vi "ORCA External Trigger with Piezo.vi"() -> ()   [LabVIEW 2012]
uses:
  <vilib>/DAQmx/write.llb/DAQmx Write (Digital Bool 1Line 1Point).vi
  <vilib>/DAQmx/create/channels.llb/DAQmx Create Channel (DO-Digital Output).vi
  <vilib>/DAQmx/write.llb/DAQmx Write (Analog DBL 1Chan 1Samp).vi
  <vilib>/DAQmx/write.llb/DAQmx Write (Digital 1D Bool 1Chan 1Samp).vi
  <vilib>/DAQmx/read.llb/DAQmx Read (Digital Bool 1Line 1Point).vi
  <vilib>/DAQmx/create/channels.llb/DAQmx Create Channel (AO-Voltage-Basic).vi
  <vilib>/DAQmx/read.llb/DAQmx Read (Analog DBL 1Chan 1Samp).vi
  <vilib>/DAQmx/create/channels.llb/DAQmx Create Channel (AI-Voltage-Basic).vi
  <vilib>/Instr/_visa.llb/VISA Configure Serial Port (Instr).vi
  <vilib>/DAQmx/create/channels.llb/DAQmx Create Channel (DI-Digital Input).vi
panel:
  out "Time to next":dbl
  out "Last pos":bool
  out "Waiting":bool
  out "First pos":bool
  out "Pos N":i32
  in  "Positions":i32=1 min=0 max=50 step=1
  in  "Next Pos":bool
  in  "Manual LCVR?":bool
  in  "z offset (um)":dbl=0.29
  in  "use z offset":bool
  in  "Auto Z":bool
  out "Z move":bool
  out "z #":i16
  in  "z step (um)":dbl=0.01
  in  "# z steps":i16=1
  in  "Piezo (um)":dbl format="%#_4g"
  in  "Piezo V":dbl min=0.0 max=10.0 step=0.01 format="%_4g"
  out "Output V":dbl
  in  "Voltages":dbl[][](array[numeric])=[[6.1, 5.6], [1.9, 2.4], [3.3, 3.6]] min=0.0 max=8.0 step=0.1 format="%0.3f"
  in  "LCVR V":dbl min=0.0 max=8.0 step=0.2
  in  "Manual DIO":bool
  in  "Live mode":bool
  out "Duration (s)":dbl
  in  "Int unit":enum16{"ms", "s", "min"}(ring)
  in  "Interval":u32 max=1000 step=1
  in  "Stop acq":bool
  in  "Exposure (ms)":u32=50 min=1 max=2000 step=5
  out "Ch N":T1
  in  "Ch 2":T2(radio)=enum."Radio Selection 3"
  out "Ch":enum32{"0", "1", "2"}(radio)
  in  "Ch 1":T2(radio)=enum."Radio Selection 2"
  in  "Ch 0":T2(radio)
  out "Current Frame":i32
  out "Total Frames":i16
  in  "Frames":i16=1
  in  "Channels":i16=1 min=1 max=3 step=1
  in  "SIM \nFrames":i16=9
  in  "stop":bool
  in  "Acquire":bool
  # "LCVR Voltage Settings"
  # "Voltage #"
  # "Channel #"
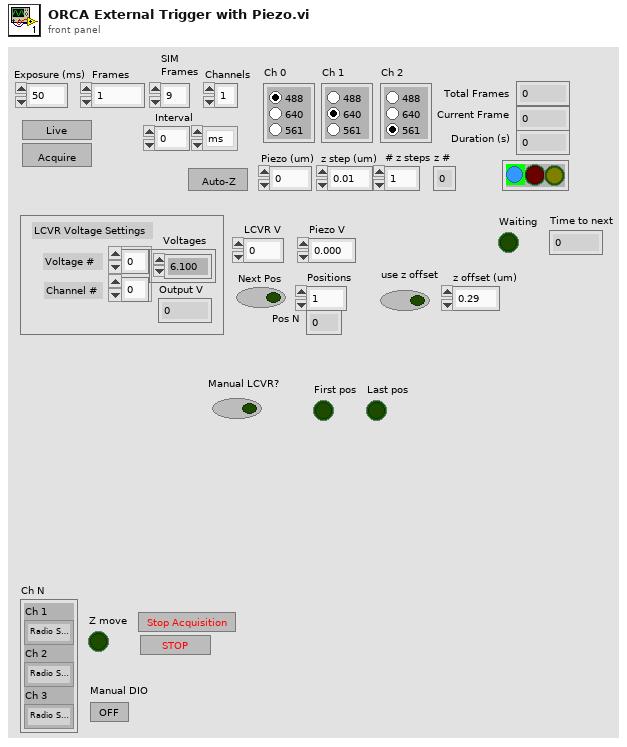
[diagram p1: front panel]
types:
  T1 = cluster{"Ch 1":enum32{"Radio Selection 1", "Radio Selection 2", "Radio Selection 3"}, "Ch 2":enum32{"Radio Selection 1", "Radio Selection 2", "Radio Selection 3"}, "Ch 3":enum32{"Radio Selection 1", "Radio Selection 2", "Radio Selection 3"}}
  T2 = enum32{"Radio Selection 1", "Radio Selection 2", "Radio Selection 3"}
  T3 = cluster{"Ch 0":enum32{"Radio Selection 1", "Radio Selection 2", "Radio Selection 3"}, "Ch 1":enum32{"Radio Selection 1", "Radio Selection 2", "Radio Selection 3"}, "Ch 2":enum32{"Radio Selection 1", "Radio Selection 2", "Radio Selection 3"}}
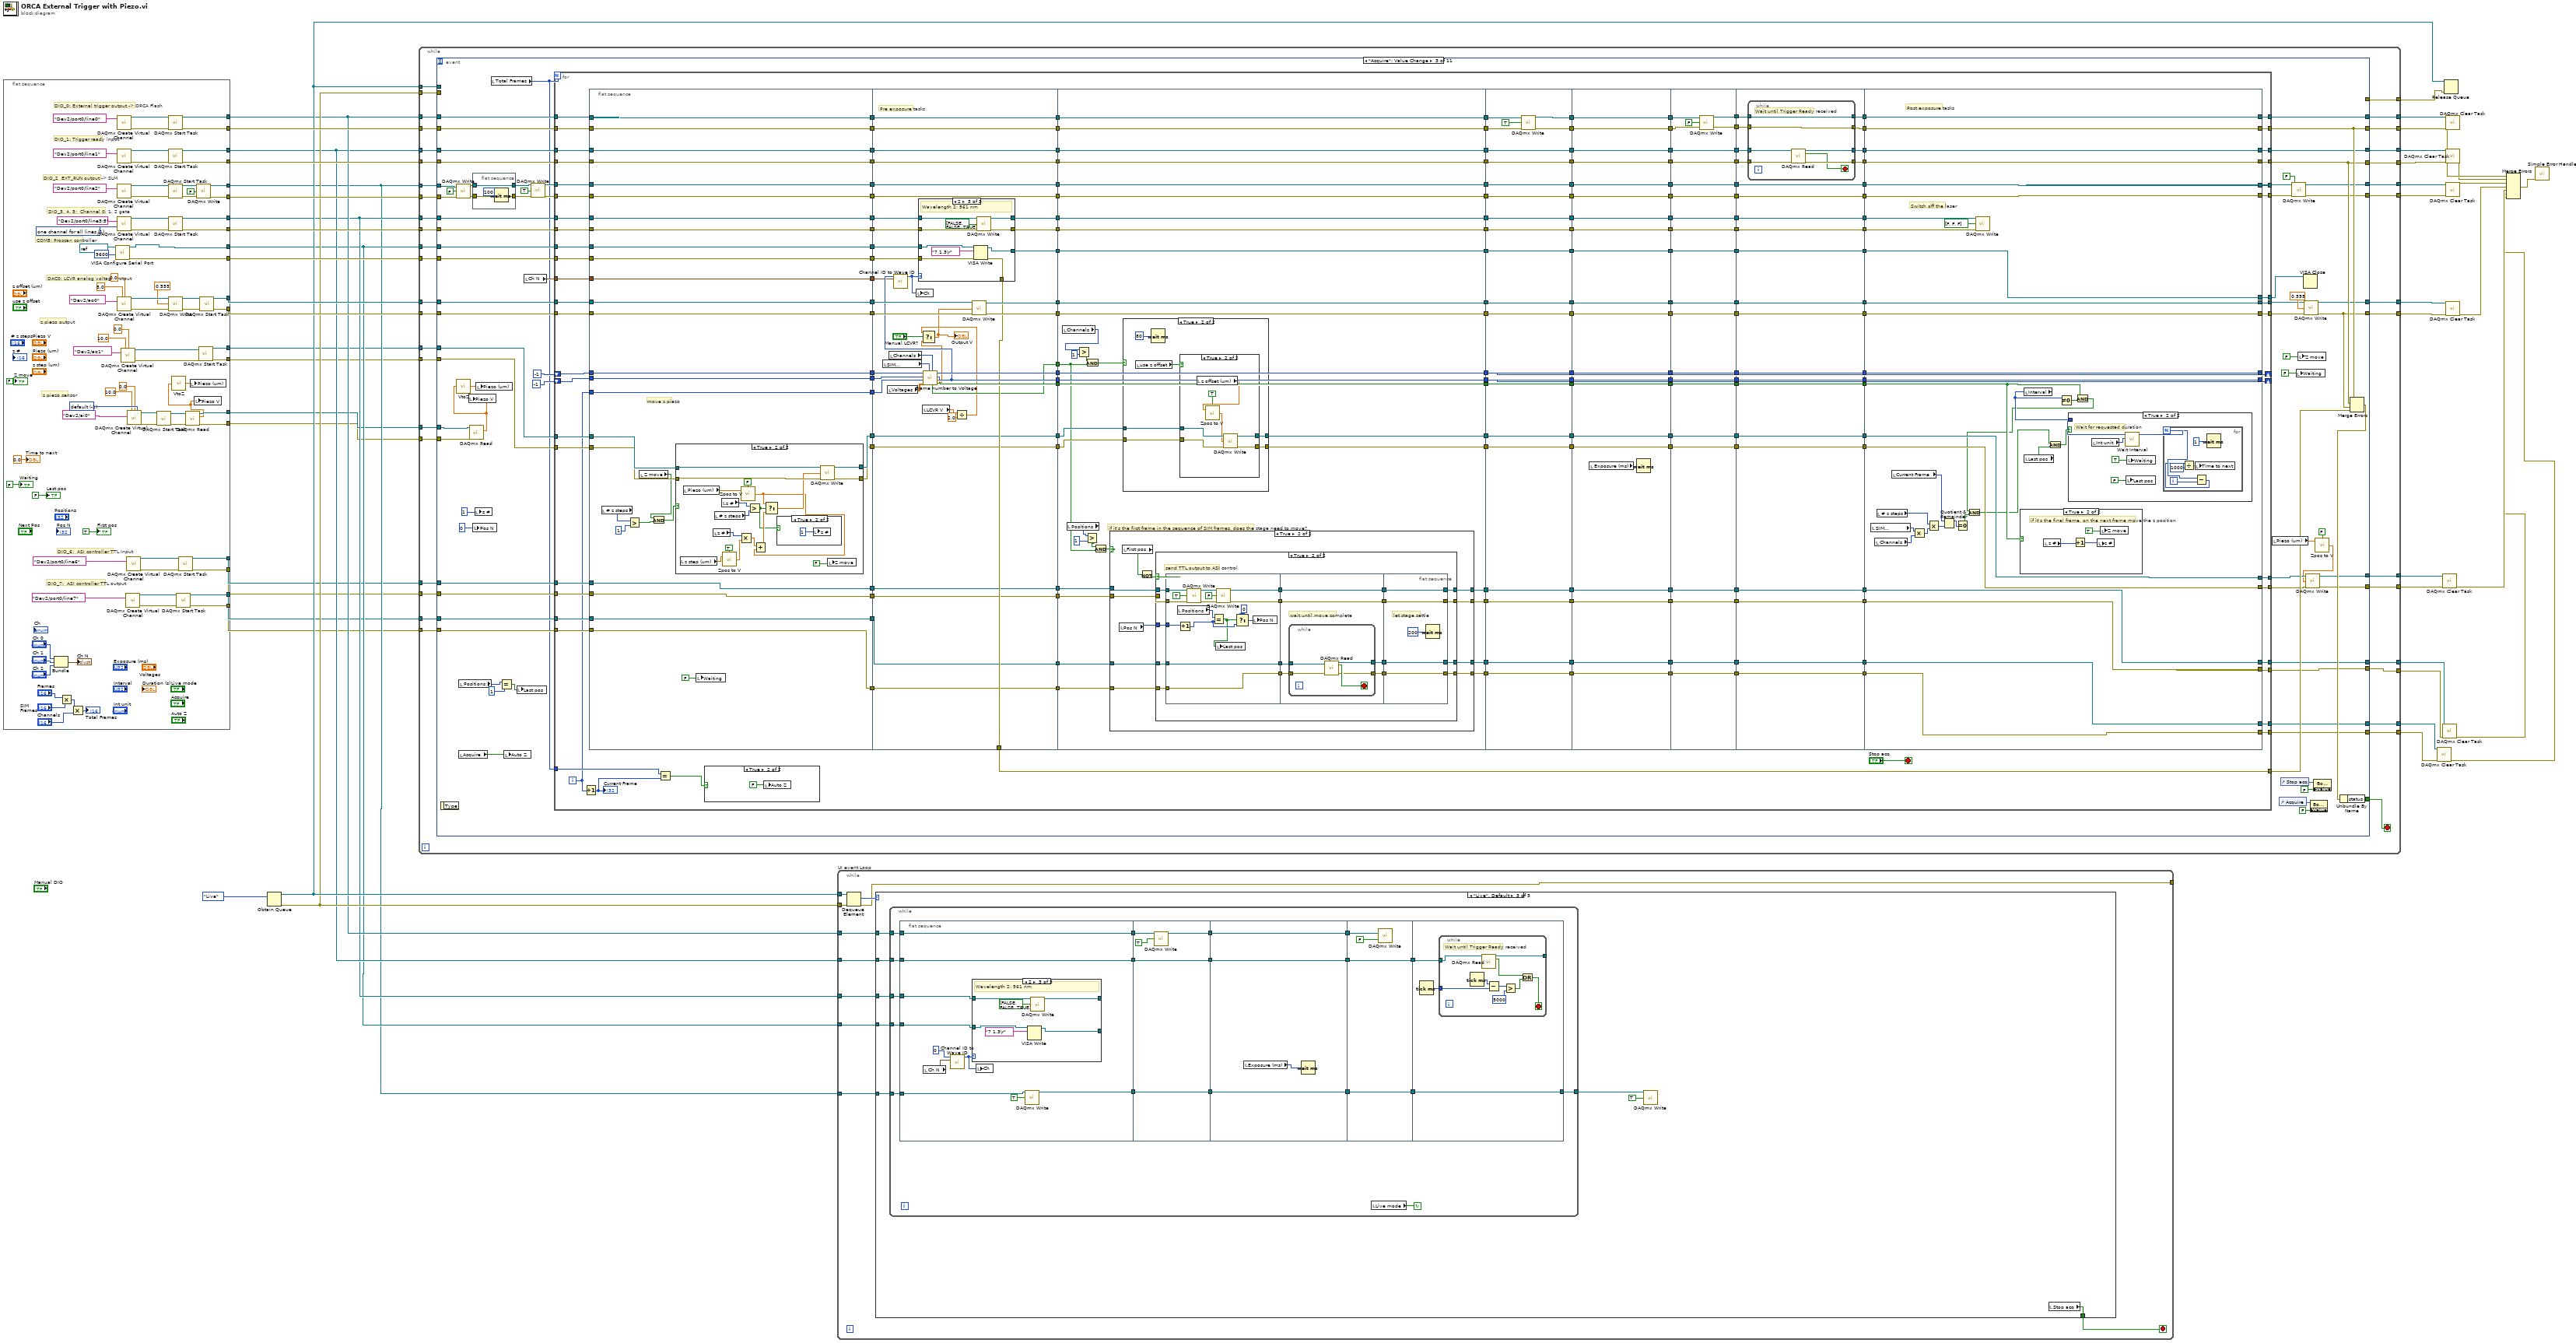
[diagram p0: block diagram]
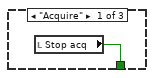
[diagram p2: hidden frame]
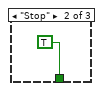
[diagram p3: hidden frame]
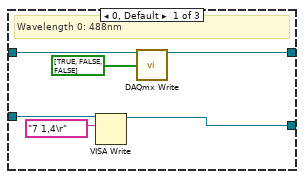
[diagram p4: hidden frame]
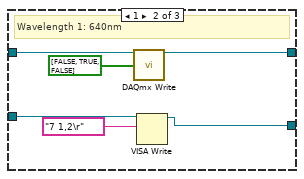
[diagram p5: hidden frame]
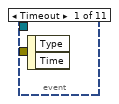
[diagram p6: hidden frame]
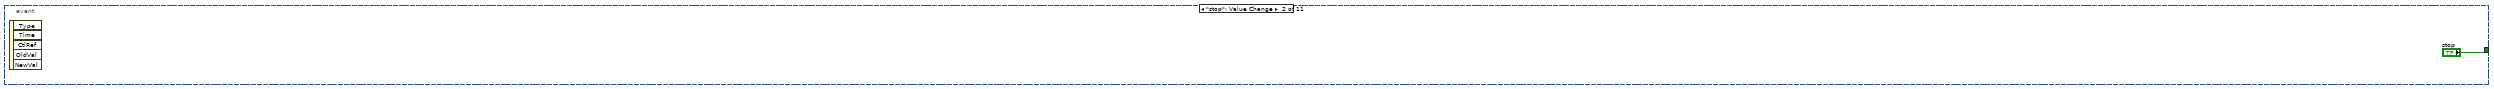
[diagram p7: hidden frame]
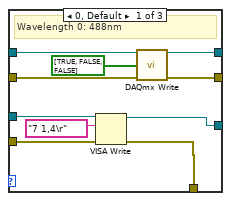
[diagram p11: hidden frame]
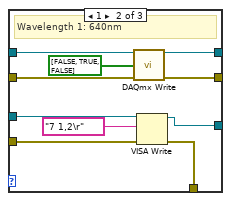
[diagram p12: hidden frame]
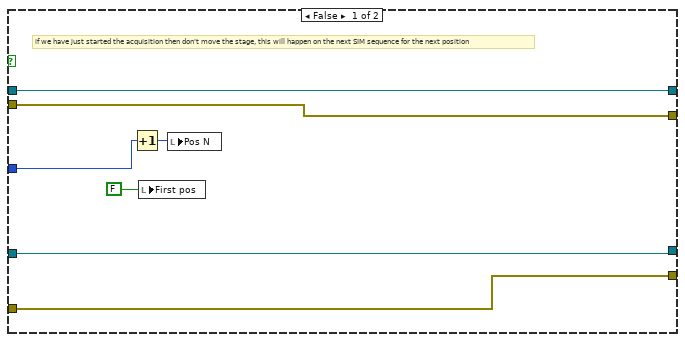
[diagram p14: hidden frame]
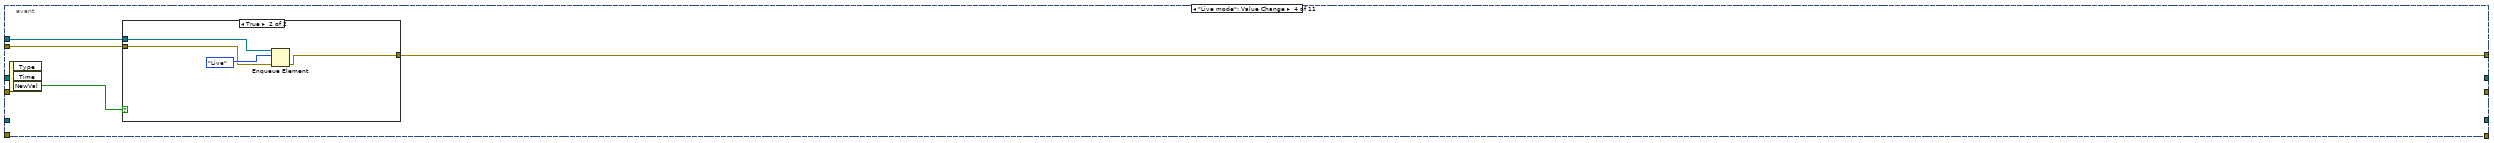
[diagram p19: hidden frame]
diagram:
  n1 = flat-sequence {
    tunnel: [w124] -> w22
    tunnel: [w123] -> w45
    tunnel: [w119] -> w21
    tunnel: [w118] -> w43
    tunnel: [w104] -> w40
    tunnel: [w103] -> w39
    tunnel: [w94] -> w18
    tunnel: [w93] -> w33
    tunnel: [w92] -> w20
    tunnel: [w91] -> w28
    tunnel: [w82] -> w19
    tunnel: [w81] -> w27
    tunnel: [w64] -> w17
    tunnel: [w65] -> w16
    tunnel: [w71] -> w15
    tunnel: [w70] -> w14
    tunnel: [w57] -> w10
    tunnel: [w56] -> w9
    tunnel: [w51] -> w5
    tunnel: [w50] -> w4
    frame #0 {
      w74 = -1 items=["default"=-1, "RSE"=10083, "NRSE"=10078, "Differential"=10106, "Pseudodifferential"=12529] ("input terminal configuration")
      w89 = 1 items=["one channel for each line", "one channel for all lines"] ("line grouping")
      # "DIO_7:  ASI controller TTL output"
      # "DIO_6:  ASI controller TTL Input"
      # "z piezo sensor"
      # "z piezo output"
      # "COM5: Proscan controller"
      # "DIO_3, 4, 5:  Channel 0, 1, 2 gate"
      # "DIO_2  EXT_RUN output -> SLM"
      # "DAC0: LCVR analog voltage output"
      # "DIO_1: Trigger ready input"
      # "DIO_0: External trigger output -> ORCA Flash"
      n2 = Bundle("Ch 0"="Ch 0", "Ch 1"="Ch 1", "Ch 2"="Ch 2") -> (→"Ch N":T3)  [unwired: 1 in]
      n3 = Multiply(x="Frames", y="SIM \nFrames") -> (x*y=w115:i16)
      n4 = Multiply(x=w115, y="Channels") -> (x*y=→"Total Frames":i16)
      n5 = call-poly "VISA Configure Serial Port"("VISA resource name"=refnum<visa-resource-name> "COM5", "baud rate (9600)"=u32 9600) -> ("VISA resource name out"=w82:refnum<visa-resource-name>, "error out"=w81:errorcluster)  [unwired: 12 in]
      n6 = call-poly <vilib>:"DAQmx Create Virtual Channel.vi"("lines"=tag "Dev2/port0/line0") -> ("task out"=w126:refnum<k21>, "error out"=w127:errorcluster)  [unwired: 13 in]
      n7 = call-poly <vilib>:"DAQmx Create Virtual Channel.vi"("lines"=tag "Dev2/port0/line1") -> ("task out"=w121:refnum<k21>, "error out"=w120:errorcluster)  [unwired: 13 in]
      n8 = call-poly <vilib>:"DAQmx Create Virtual Channel.vi"("lines"=tag "Dev2/port0/line2") -> ("task out"=w101:refnum<k21>, "error out"=w100:errorcluster)  [unwired: 13 in]
      n9 = call-poly <vilib>:"DAQmx Create Virtual Channel.vi"("lines"="Dev2/port0/line3:5", "line grouping"=w89) -> ("task out"=w99:refnum<k21>, "error out"=w98:errorcluster)  [unwired: 12 in]
      n10 = call-poly <vilib>:"DAQmx Create Virtual Channel.vi"("maximum value"=5.0, "minimum value"=0.0, "physical channels"=tag "Dev2/ao0") -> ("task out"=w107:refnum<k21>, "error out"=w106:errorcluster)  [unwired: 11 in]
      n11 = call-poly <vilib>:"DAQmx Create Virtual Channel.vi"("maximum value"=10.0, "minimum value"=0.0, "physical channels"=tag "Dev2/ao1") -> ("task out"=w77:refnum<k21>, "error out"=w76:errorcluster)  [unwired: 11 in]
      n12 = call-poly <vilib>:"DAQmx Create Virtual Channel.vi"("lines"=tag "Dev2/port0/line7") -> ("task out"=w53:refnum<k21>, "error out"=w52:errorcluster)  [unwired: 13 in]
      n13 = call-poly <vilib>:"DAQmx Create Virtual Channel.vi"("lines"=tag "Dev2/port0/line6") -> ("task out"=w59:refnum<k21>, "error out"=w58:errorcluster)  [unwired: 13 in]
      n14 = call-poly <vilib>:"DAQmx Create Virtual Channel.vi"("maximum value"=10.0, "minimum value"=0.0, "input terminal configuration"=w74, "physical channels"=tag "Dev2/ai0" ("Physical Channel")) -> ("task out"=w69:refnum<k21>, "error out"=w68:errorcluster)  [unwired: 10 in]
      n15 = call <vilib>:"DAQmx Start Task.vi"("task/channels in"=w69, "error in"=w68) -> ("task out"=w67:refnum<k21>, "error out"=w66:errorcluster)  [unwired: 12 in]
      n16 = call <vilib>:"DAQmx Start Task.vi"("task/channels in"=w126, "error in"=w127) -> ("task out"=w124:refnum<k21>, "error out"=w123:errorcluster)  [unwired: 12 in]
      n17 = call <vilib>:"DAQmx Start Task.vi"("task/channels in"=w121, "error in"=w120) -> ("task out"=w119:refnum<k21>, "error out"=w118:errorcluster)  [unwired: 12 in]
      n18 = call <vilib>:"DAQmx Start Task.vi"("task/channels in"=w101, "error in"=w100) -> ("task out"=w97:refnum<k21>, "error out"=w96:errorcluster)  [unwired: 12 in]
      n19 = call <vilib>:"DAQmx Start Task.vi"("task/channels in"=w99, "error in"=w98) -> ("task out"=w92:refnum<k21>, "error out"=w91:errorcluster)  [unwired: 12 in]
      n20 = call-poly <vilib>:"DAQmx Write.vi"("task/channels in"=w107, "data"=0.555, "error in"=w106) -> ("task out"=w111:refnum<k21>, "error out"=w110:errorcluster)  [unwired: 10 in, 1 out]
      n21 = call <vilib>:"DAQmx Start Task.vi"("task/channels in"=w53, "error in"=w52) -> ("task out"=w51:refnum<k21>, "error out"=w50:errorcluster)  [unwired: 12 in]
      n22 = call <vilib>:"DAQmx Start Task.vi"("task/channels in"=w59, "error in"=w58) -> ("task out"=w57:refnum<k21>, "error out"=w56:errorcluster)  [unwired: 12 in]
      n23 = call-poly <vilib>:"DAQmx Read.vi"("task/channels in"=w67, "error in"=w66) -> ("task out"=w64:refnum<k21>, "data"=w61:dbl, "error out"=w65:errorcluster)  [unwired: 11 in]
      n24 = call "VtoZ.vi"("Voltage IN"=w61) -> ("Zpos OUT (um)"=w62:dbl)
      n25 = local write "Piezo (um)"(w62) -> ()
      n26 = local write "Piezo V"(w61) -> ()
      n27 = call-poly <vilib>:"DAQmx Write.vi"("task/channels in"=w97, "data"=FALSE, "error in"=w96) -> ("task out"=w94:refnum<k21>, "error out"=w93:errorcluster)  [unwired: 10 in, 1 out]
      n28 = call <vilib>:"DAQmx Start Task.vi"("task/channels in"=w77, "error in"=w76) -> ("task out"=w71:refnum<k21>, "error out"=w70:errorcluster)  [unwired: 12 in]
      n29 = call <vilib>:"DAQmx Start Task.vi"("task/channels in"=w111, "error in"=w110) -> ("task out"=w104:refnum<k21>, "error out"=w103:errorcluster)  [unwired: 12 in]
      "Z move" <- FALSE ("Z move")
      "First pos" <- TRUE ("First pos")
      "Waiting" <- FALSE ("Waiting")
      "Last pos" <- FALSE ("Last pos")
      "Time to next" <- 0.0 ("Time to next")
    }
  }
  n30 = Obtain Queue(element data type=enum16{"Live", "Stop", "Acquire"}."Live") -> (queue out=w25:refnum<queue>, error out=w23:errorcluster)  [unwired: 4 in, 1 out]
  n31 = while {
    tunnel: w22 -> [w164]
    tunnel: [w163] -> w46
    tunnel: w45 -> [w162]
    tunnel: [w161] -> w44
    tunnel: w21 -> [w160]
    tunnel: w43 -> [w159]
    tunnel: [w158] -> w42
    tunnel: [w157] -> w41
    tunnel: w40 -> [w156]
    tunnel: w39 -> [w155]
    tunnel: [w154] -> w35
    tunnel: [w153] -> w34
    tunnel: w18 -> [w152]
    tunnel: w33 -> [w151]
    tunnel: [w150] -> w29
    tunnel: [w149] -> w31
    tunnel: w20 -> [w148]
    tunnel: w28 -> [w147]
    tunnel: w19 -> [w146]
    tunnel: w27 -> [w145]
    tunnel: w25 -> [w144]
    tunnel: [w143] -> w24
    tunnel: w23 -> [w142]
    tunnel: w17 -> [w141]
    tunnel: w16 -> [w140]
    tunnel: w15 -> [w139]
    tunnel: w14 -> [w138]
    tunnel: [w137] -> w13
    tunnel: [w136] -> w12
    tunnel: w10 -> [w135]
    tunnel: w9 -> [w134]
    tunnel: [w133] -> w7
    tunnel: [w132] -> w6
    tunnel: w5 -> [w131]
    tunnel: w4 -> [w130]
    tunnel: [w129] -> w2
    tunnel: [w128] -> w1
    stop <- w165 stop-if-true
    n32 = event shown="[2] \"Acquire\": Value Change" {
      selector: _ -> [_ _ _ _ _ _ _ _ _ _ _]
      dyn-events: _ -> [_ _ _ _ _ _ _ _ _ _ _]
      timeout: _ -> [_ _ _ _ _ _ _ _ _ _ _]
      tunnel: [_ "stop" w241 _ _ _ _ _ _ _ _] -> w165
      tunnel: w164 -> [_ _ w240 _ _ _ _ _ _ _ _]
      tunnel: [_ _ w238 _ _ _ _ _ _ _ _] -> w163
      tunnel: w162 -> [_ _ w239 _ _ _ _ _ _ _ _]
      tunnel: [_ _ w232 _ _ _ _ _ _ _ _] -> w161
      tunnel: w160 -> [_ _ w235 _ _ _ _ _ _ _ _]
      tunnel: w159 -> [_ _ w234 _ _ _ _ _ _ _ _]
      tunnel: [_ _ w231 _ _ _ _ _ _ _ _] -> w158
      tunnel: [_ _ w230 _ _ _ _ _ _ _ _] -> w157
      tunnel: w156 -> [_ _ w227 _ _ w858 _ _ _ _ _]
      tunnel: w155 -> [_ _ w226 _ _ w857 _ _ _ _ _]
      tunnel: [_ _ w222 _ _ _ _ _ _ _ _] -> w154
      tunnel: [_ _ w221 _ _ _ _ _ _ _ _] -> w153
      tunnel: w152 -> [_ _ w202 _ _ _ _ _ _ _ _]
      tunnel: w151 -> [_ _ w201 _ _ _ _ _ _ _ _]
      tunnel: [_ _ w204 _ _ _ _ _ _ _ _] -> w150
      tunnel: [_ _ w206 _ _ _ _ _ _ _ _] -> w149
      tunnel: w148 -> [_ _ w217 _ w838 _ _ _ _ _ _]
      tunnel: w147 -> [_ _ w216 _ w837 _ _ _ _ _ _]
      tunnel: w146 -> [_ _ w212 _ _ _ _ _ _ _ _]
      tunnel: w145 -> [_ _ w211 _ _ _ _ _ _ _ _]
      tunnel: w144 -> [_ _ _ w827 _ _ _ _ _ _ _]
      tunnel: [_ _ _ w826 _ _ _ _ _ _ _] -> w143
      tunnel: w142 -> [_ _ _ w825 _ _ _ _ _ _ _]
      tunnel: w141 -> [_ _ w196 _ _ _ _ _ _ w893 _]
      tunnel: w140 -> [_ _ w195 _ _ _ _ _ _ w892 _]
      tunnel: w139 -> [_ _ w194 _ _ _ _ _ w885 w891 _]
      tunnel: w138 -> [_ _ w193 _ _ _ _ _ w884 w888 _]
      tunnel: [_ _ w188 _ _ _ _ _ _ _ _] -> w137
      tunnel: [_ _ w187 _ _ _ _ _ _ _ _] -> w136
      tunnel: w135 -> [_ _ w181 _ _ _ _ _ _ _ w913]
      tunnel: w134 -> [_ _ w180 _ _ _ _ _ _ _ w912]
      tunnel: [_ _ w178 _ _ _ _ _ _ _ _] -> w133
      tunnel: [_ _ w177 _ _ _ _ _ _ _ _] -> w132
      tunnel: w131 -> [_ _ w176 _ _ _ _ _ _ _ _]
      tunnel: w130 -> [_ _ w175 _ _ _ _ _ _ _ _]
      tunnel: [_ _ w174 _ _ _ _ _ _ _ _] -> w129
      tunnel: [_ _ w173 _ _ _ _ _ _ _ _] -> w128
      event Timeout {
        n33 = event-data() -> ()  [unwired: 1 in, 2 out]
      }
      event "stop": Value Change {
        n34 = event-data() -> ()  [unwired: 1 in, 5 out]
      }
      event "Acquire": Value Change {
        n35 = event-data() -> ()  [unwired: 1 in, 1 out]
        n36 = call-poly <vilib>:"DAQmx Write.vi"("task/channels in"=w202, "data"=FALSE, "error in"=w201) -> ("task out"=w197:refnum<k21>, "error out"=w199:errorcluster)  [unwired: 10 in, 1 out]
        n37 = local read "Acquire"() -> (w168:bool)
        n38 = local read "Positions"() -> (w171:i32)
        n39 = call-poly <vilib>:"DAQmx Read.vi"("task/channels in"=w196, "error in"=w195) -> ("data"=w185:dbl)  [unwired: 11 in, 2 out]
        n40 = call "VtoZ.vi"("Voltage IN"=w185) -> ("Zpos OUT (um)"=w186:dbl)
        n41 = local write "Piezo V"(w185) -> ()
        n42 = local write "Pos N"(0 ("Pos N")) -> ()
        n43 = flat-sequence {
          tunnel: [w244] -> w200
          tunnel: w199 -> [w244]
          tunnel: [w243] -> w198
          tunnel: w197 -> [w243]
          frame #0 {
            n44 = Wait (ms)(milliseconds to wait=u32 100) -> ()  [unwired: 1 out]
          }
        }
        n45 = local write "z #"(i16 1 ("z #")) -> ()
        n46 = local write "Piezo (um)"(w186) -> ()
        n47 = local read "Total Frames"() -> (w167:i16)
        n48 = Equal?(x=w171, y=1) -> (x = y?=w169:bool)
        n49 = local write "Auto Z"(w168) -> ()
        n50 = local write "Last pos"(w169) -> ()
        n51 = local read "Ch N"() -> (w215:T1)
        n52 = call-poly <vilib>:"DAQmx Write.vi"("task/channels in"=w198, "data"=TRUE, "error in"=w200) -> ("task out"=w219:refnum<k21>, "error out"=w218:errorcluster)  [unwired: 10 in, 1 out]
        n53 = for {
          N: w167 -> [_]
          tunnel: w240 -> [w431]
          tunnel: w239 -> [w430]
          tunnel: [w428] -> w238
          tunnel: [w427] -> w232
          tunnel: w235 -> [w425]
          tunnel: w234 -> [w423]
          tunnel: [w422] -> w231
          tunnel: [w421] -> w230
          shift-right: [w417] -> _
          shift-left: i16 -1 ("Voltage out") -> [w419]
          shift-right: [w415] -> _
          shift-left: i16 -1 ("Channel out") -> [w418]
          tunnel: w227 -> [w413]
          tunnel: w226 -> [w412]
          tunnel: [w411] -> w224
          tunnel: [w409] -> w223
          tunnel: [w399] -> w207
          tunnel: w219 -> [w396]
          tunnel: [w395] -> w205
          tunnel: w218 -> [w392]
          tunnel: w217 -> [w391]
          tunnel: w216 -> [w390]
          tunnel: w215 -> [w389]
          tunnel: w212 -> [w355]
          tunnel: w211 -> [w354]
          tunnel: [w353] -> w209
          tunnel: [w348] -> w210
          tunnel: w194 -> [w302]
          tunnel: w193 -> [w301]
          tunnel: [w293] -> w190
          tunnel: [w289] -> w189
          tunnel: w181 -> [w284]
          tunnel: w180 -> [w283]
          tunnel: [w268] -> w178
          tunnel: [w267] -> w177
          tunnel: w176 -> [w266]
          tunnel: w175 -> [w265]
          tunnel: [w250] -> w174
          tunnel: [w249] -> w173
          tunnel: w167 -> [w248]
          i -> [w246]
          stop <- "Stop acq" stop-if-true
          n54 = Increment(x=w246) -> (x+1=w245:i32)
          "Current Frame" <- w245
          n55 = flat-sequence {
            tunnel: w354 -> [w447]
            tunnel: w355 -> [w448]
            tunnel: w389 -> [w449]
            tunnel: w390 -> [w450]
            tunnel: w391 -> [w451]
            tunnel: w392 -> [w452]
            tunnel: w396 -> [w453]
            tunnel: w412 -> [w454]
            tunnel: w413 -> [w455]
            tunnel: w418 -> [w456]
            tunnel: w419 -> [w457]
            tunnel: w246 -> [w458]
            tunnel: w423 -> [w459]
            tunnel: w425 -> [w460]
            tunnel: w430 -> [w461]
            tunnel: w431 -> [w462]
            tunnel: [w462] -> w318
            tunnel: [w461] -> w317
            tunnel: [w460] -> w316
            tunnel: [w459] -> w315
            tunnel: [w458] -> w314
            tunnel: [w457] -> w313
            tunnel: [w456] -> w312
            tunnel: [w455] -> w311
            tunnel: [w454] -> w310
            tunnel: [w453] -> w309
            tunnel: [w452] -> w308
            tunnel: [w451] -> w307
            tunnel: [w450] -> w306
            tunnel: [w449] -> w305
            tunnel: [w448] -> w304
            tunnel: [w447] -> w303
            tunnel: w302 -> [w446]
            tunnel: w301 -> [w445]
            tunnel: [w439] -> w297
            tunnel: [w438] -> w294
            tunnel: w284 -> [w437]
            tunnel: w283 -> [w436]
            tunnel: [w437] -> w281
            tunnel: [w436] -> w279
            tunnel: w266 -> [w435]
            tunnel: w265 -> [w434]
            tunnel: [w435] -> w263
            tunnel: [w434] -> w261
            tunnel: [w525] -> w347
            tunnel: [w524] -> w345
            tunnel: [w523] -> w343
            tunnel: [w522] -> w341
            tunnel: [w516] -> w339
            tunnel: [w506] -> w337
            tunnel: [w512] -> w335
            tunnel: [w511] -> w333
            tunnel: [w510] -> w331
            tunnel: [w509] -> w329
            tunnel: [w503] -> w327
            tunnel: [w502] -> w325
            tunnel: [w501] -> w323
            tunnel: [w498] -> w321
            tunnel: [w497] -> w348
            tunnel: [w496] -> w319
            tunnel: w318 -> [w525]
            tunnel: w317 -> [w524]
            tunnel: w316 -> [w523]
            tunnel: w315 -> [w522]
            tunnel: w314 -> [w517]
            tunnel: w313 -> [w519]
            tunnel: w312 -> [w518]
            tunnel: w311 -> [w514]
            tunnel: w310 -> [w513]
            tunnel: w309 -> [w510]
            tunnel: w308 -> [w509]
            tunnel: w307 -> [w508]
            tunnel: w306 -> [w507]
            tunnel: w305 -> [w504]
            tunnel: w304 -> [w500]
            tunnel: w303 -> [w499]
            tunnel: [w495] -> w298
            tunnel: w297 -> [w495]
            tunnel: [w494] -> w295
            tunnel: w294 -> [w494]
            tunnel: [w487] -> w282
            tunnel: w281 -> [w487]
            tunnel: [w486] -> w280
            tunnel: w279 -> [w486]
            tunnel: [w485] -> w264
            tunnel: w263 -> [w485]
            tunnel: [w484] -> w262
            tunnel: w261 -> [w484]
            tunnel: w347 -> [w590]
            tunnel: [w590] -> w346
            tunnel: w345 -> [w589]
            tunnel: [w589] -> w344
            tunnel: w343 -> [w588]
            tunnel: [w588] -> w342
            tunnel: w341 -> [w587]
            tunnel: [w587] -> w340
            tunnel: w339 -> [w586]
            tunnel: [w586] -> w338
            tunnel: w337 -> [w585]
            tunnel: [w585] -> w336
            tunnel: w335 -> [w584]
            tunnel: [w584] -> w334
            tunnel: w333 -> [w583]
            tunnel: [w583] -> w332
            tunnel: w331 -> [w582]
            tunnel: [w582] -> w330
            tunnel: w329 -> [w581]
            tunnel: [w581] -> w328
            tunnel: w327 -> [w580]
            tunnel: [w580] -> w326
            tunnel: w325 -> [w579]
            tunnel: [w579] -> w324
            tunnel: w323 -> [w578]
            tunnel: [w578] -> w322
            tunnel: w321 -> [w577]
            tunnel: [w577] -> w320
            tunnel: w319 -> [w568]
            tunnel: [w570] -> w299
            tunnel: w298 -> [w572]
            tunnel: w295 -> [w571]
            tunnel: [w569] -> w285
            tunnel: w282 -> [w564]
            tunnel: w280 -> [w563]
            tunnel: [w561] -> w274
            tunnel: [w560] -> w269
            tunnel: w264 -> [w559]
            tunnel: w262 -> [w558]
            tunnel: [w557] -> w256
            tunnel: [w556] -> w251
            tunnel: [w698] -> w388
            tunnel: [w697] -> w386
            tunnel: [w696] -> w384
            tunnel: [w695] -> w382
            tunnel: w346 -> [w700]
            tunnel: w344 -> [w699]
            tunnel: w342 -> [w696]
            tunnel: w340 -> [w695]
            tunnel: [w694] -> w380
            tunnel: w338 -> [w694]
            tunnel: [w693] -> w378
            tunnel: w336 -> [w693]
            tunnel: [w692] -> w376
            tunnel: w334 -> [w692]
            tunnel: [w691] -> w374
            tunnel: w332 -> [w691]
            tunnel: [w690] -> w372
            tunnel: w330 -> [w690]
            tunnel: [w689] -> w370
            tunnel: w328 -> [w689]
            tunnel: [w688] -> w364
            tunnel: w326 -> [w688]
            tunnel: [w687] -> w360
            tunnel: w324 -> [w687]
            tunnel: [w686] -> w356
            tunnel: w322 -> [w686]
            tunnel: [w685] -> w349
            tunnel: w320 -> [w685]
            tunnel: [w684] -> w300
            tunnel: w299 -> [w684]
            tunnel: [w683] -> w296
            tunnel: w285 -> [w683]
            tunnel: [w682] -> w275
            tunnel: w274 -> [w682]
            tunnel: [w681] -> w270
            tunnel: w269 -> [w681]
            tunnel: [w680] -> w257
            tunnel: w256 -> [w680]
            tunnel: [w679] -> w252
            tunnel: w251 -> [w679]
            tunnel: w388 -> [w722]
            tunnel: [w722] -> w387
            tunnel: w386 -> [w721]
            tunnel: [w721] -> w385
            tunnel: w384 -> [w720]
            tunnel: [w720] -> w383
            tunnel: w382 -> [w719]
            tunnel: [w719] -> w381
            tunnel: w380 -> [w718]
            tunnel: [w718] -> w379
            tunnel: w378 -> [w717]
            tunnel: [w717] -> w377
            tunnel: w376 -> [w716]
            tunnel: [w716] -> w375
            tunnel: w374 -> [w715]
            tunnel: [w715] -> w373
            tunnel: w372 -> [w714]
            tunnel: [w714] -> w371
            tunnel: w370 -> [w713]
            tunnel: [w713] -> w369
            tunnel: [w712] -> w365
            tunnel: w364 -> [w712]
            tunnel: [w711] -> w361
            tunnel: w360 -> [w711]
            tunnel: [w710] -> w357
            tunnel: w356 -> [w710]
            tunnel: [w709] -> w350
            tunnel: w349 -> [w709]
            tunnel: w300 -> [w708]
            tunnel: w296 -> [w707]
            tunnel: [w708] -> w290
            tunnel: [w707] -> w286
            tunnel: [w705] -> w276
            tunnel: w275 -> [w705]
            tunnel: [w704] -> w271
            tunnel: w270 -> [w704]
            tunnel: [w703] -> w258
            tunnel: w257 -> [w703]
            tunnel: [w702] -> w253
            tunnel: w252 -> [w702]
            tunnel: w387 -> [w739]
            tunnel: [w744] -> w429
            tunnel: w385 -> [w744]
            tunnel: [w743] -> w426
            tunnel: w383 -> [w743]
            tunnel: [w742] -> w424
            tunnel: w381 -> [w742]
            tunnel: [w740] -> w420
            tunnel: [w738] -> w416
            tunnel: w379 -> [w738]
            tunnel: [w737] -> w414
            tunnel: w377 -> [w737]
            tunnel: [w736] -> w410
            tunnel: w375 -> [w736]
            tunnel: [w735] -> w408
            tunnel: w373 -> [w735]
            tunnel: [w734] -> w397
            tunnel: w371 -> [w734]
            tunnel: [w733] -> w393
            tunnel: w369 -> [w733]
            tunnel: [w732] -> w366
            tunnel: w365 -> [w732]
            tunnel: [w731] -> w362
            tunnel: w361 -> [w731]
            tunnel: [w730] -> w358
            tunnel: w357 -> [w730]
            tunnel: [w729] -> w351
            tunnel: w350 -> [w729]
            tunnel: [w728] -> w291
            tunnel: w290 -> [w728]
            tunnel: [w727] -> w287
            tunnel: w286 -> [w727]
            tunnel: [w726] -> w277
            tunnel: w276 -> [w726]
            tunnel: [w725] -> w272
            tunnel: w271 -> [w725]
            tunnel: [w724] -> w259
            tunnel: w258 -> [w724]
            tunnel: [w723] -> w254
            tunnel: w253 -> [w723]
            tunnel: w429 -> [w765]
            tunnel: w426 -> [w764]
            tunnel: w424 -> [w763]
            tunnel: w420 -> [w767]
            tunnel: w416 -> [w760]
            tunnel: w414 -> [w759]
            tunnel: w410 -> [w758]
            tunnel: w408 -> [w757]
            tunnel: [w768] -> w407
            tunnel: [w766] -> w406
            tunnel: [w762] -> w405
            tunnel: [w761] -> w404
            tunnel: [w760] -> w403
            tunnel: [w759] -> w402
            tunnel: [w758] -> w401
            tunnel: [w757] -> w400
            tunnel: [w756] -> w398
            tunnel: w397 -> [w756]
            tunnel: [w755] -> w394
            tunnel: w393 -> [w755]
            tunnel: [w754] -> w367
            tunnel: w366 -> [w754]
            tunnel: [w753] -> w363
            tunnel: w362 -> [w753]
            tunnel: [w752] -> w359
            tunnel: w358 -> [w752]
            tunnel: [w751] -> w352
            tunnel: w351 -> [w751]
            tunnel: [w750] -> w292
            tunnel: w291 -> [w750]
            tunnel: [w749] -> w288
            tunnel: w287 -> [w749]
            tunnel: [w748] -> w278
            tunnel: w277 -> [w748]
            tunnel: [w747] -> w273
            tunnel: w272 -> [w747]
            tunnel: [w746] -> w260
            tunnel: w259 -> [w746]
            tunnel: [w745] -> w255
            tunnel: w254 -> [w745]
            tunnel: [w803] -> w409
            tunnel: [w804] -> w411
            tunnel: [w805] -> w415
            tunnel: [w806] -> w417
            tunnel: [w807] -> w421
            tunnel: [w808] -> w422
            tunnel: [w809] -> w427
            tunnel: [w810] -> w428
            tunnel: w407 -> [w810]
            tunnel: w406 -> [w809]
            tunnel: w405 -> [w808]
            tunnel: w404 -> [w807]
            tunnel: w403 -> [w806]
            tunnel: w402 -> [w805]
            tunnel: w401 -> [w804]
            tunnel: w400 -> [w803]
            tunnel: [w802] -> w399
            tunnel: w398 -> [w802]
            tunnel: [w801] -> w395
            tunnel: w394 -> [w801]
            tunnel: w367 -> [w794]
            tunnel: w363 -> [w798]
            tunnel: w359 -> [w797]
            tunnel: [w795] -> w353
            tunnel: w352 -> [w795]
            tunnel: [w793] -> w293
            tunnel: w292 -> [w793]
            tunnel: [w792] -> w289
            tunnel: w288 -> [w792]
            tunnel: w278 -> [w782]
            tunnel: w273 -> [w781]
            tunnel: [w782] -> w268
            tunnel: [w781] -> w267
            tunnel: w260 -> [w780]
            tunnel: w255 -> [w779]
            tunnel: [w780] -> w250
            tunnel: [w779] -> w249
            frame #0 {
              # "move z piezo"
              n56 = local read "# z steps"() -> (w444:i16)
              n57 = Greater?(x=w444, y=i16 1) -> (0:w442:bool)
              n58 = local read "Z move"() -> (w441:bool)
              n59 = And(x=w441, y=w442) -> (x .and. y?=w440:bool)
              n60 = case shown="True" w440 {
                tunnel: w446 -> [w464 w482]
                tunnel: w445 -> [w463 w481]
                tunnel: [w464 w472] -> w439
                tunnel: [w463 w471] -> w438
                frame False {
                }
                frame True {
                  n61 = local read "z step (um)"() -> (w467:dbl)
                  n62 = local read "Piezo (um)"() -> (w470:dbl)
                  n63 = local read "z #"() -> (w480:i16)
                  n64 = local read "# z steps"() -> (w477:i16)
                  n65 = local read "z #"() -> (w476:i16)
                  n66 = call "Zpos to V.vi"(1:TRUE ("Z step?"), "Z (um)"=w467) -> ("V"=w466:dbl)  [unwired: 1 in]
                  n67 = Multiply(x=w480, y=w466) -> (x*y=w479:dbl)
                  n68 = call "Zpos to V.vi"(1:FALSE ("Z step?"), "Z (um)"=w470) -> ("V"=w468:dbl)  [unwired: 1 in]
                  n69 = Greater?(x=w476, y=w477) -> (0:w473:bool)
                  n70 = Add(x=w479, y=w468) -> (x+y=w475:dbl)
                  n71 = Select(t=w468, s=w473, f=w475) -> (s? t:f=w474:dbl)
                  n72 = case shown="True" w473 {
                    frame False {
                    }
                    frame True {
                      n73 = local write "z #"(i16 1 ("z #")) -> ()
                    }
                  }
                  n74 = call-poly <vilib>:"DAQmx Write.vi"("task/channels in"=w482, "data"=w474, "error in"=w481) -> ("task out"=w472:refnum<k21>, "error out"=w471:errorcluster)  [unwired: 10 in, 1 out]
                  n75 = local write "Z move"(FALSE) -> ()
                }
              }
              n76 = local write "Waiting"(FALSE ("Waiting")) -> ()
            }
            frame #1 {
              # "Pre exposure tasks"
              n77 = local read "SIM \nFrames"() -> (w520:i16)
              n78 = local read "Voltages"() -> (w515:dbl[][])
              n79 = local read "Channels"() -> (w521:i16)
              n80 = local read "LCVR V"() -> (w492:dbl)
              n81 = call "Frame number to Voltage.vi"("Channel N"=w521, "SIM Frame N"=w520, "Voltages"=w515, "Frame count"=w517, "Current Channel"=w518, "Current V"=w519) -> ("Final frame?"=w503:bool, "V"=w490:dbl, "Channel out"=w506:i16, "Voltage out"=w516:i16, "First frame?"=w496:bool)  [unwired: 1 in]
              n82 = call "Channel ID to Wave ID.vi"("Ch N"=w504, "Channel ID"=w506) -> ("Wave ID"=w505:i16)  [unwired: 9 in]
              n83 = local write "Ch"(w505) -> ()
              n84 = case shown="2" w505 {
                tunnel: w508 -> [w535 w544 w548]
                tunnel: w507 -> [w534 w543 w547]
                tunnel: [w532 w542 w550] -> w502
                tunnel: [w531 w541 w549] -> w501
                tunnel: w500 -> [w529 w540 w555]
                tunnel: w499 -> [w530 w539 w554]
                tunnel: [w527 w538 w551] -> w498
                tunnel: [w526 w537 w552] -> w497
                frame 0, Default {
                  # "Wavelength 0: 488nm"
                  n85 = VISA Write(VISA resource name=w529, write buffer="7 1,4\r", error in (no error)=w530) -> (VISA resource name out=w527:refnum<visa-resource-name>, error out=w526:errorcluster)  [unwired: 1 out]
                  n86 = call-poly <vilib>:"DAQmx Write.vi"("task/channels in"=w535, "data"=bool[] [TRUE, FALSE, FALSE], "error in"=w534) -> ("task out"=w532:refnum<k21>, "error out"=w531:errorcluster)  [unwired: 10 in, 1 out]
                }
                frame 1 {
                  # "Wavelength 1: 640nm"
                  n87 = call-poly <vilib>:"DAQmx Write.vi"("task/channels in"=w544, "data"=bool[] [FALSE, TRUE, FALSE], "error in"=w543) -> ("task out"=w542:refnum<k21>, "error out"=w541:errorcluster)  [unwired: 10 in, 1 out]
                  n88 = VISA Write(VISA resource name=w540, write buffer="7 1,2\r", error in (no error)=w539) -> (VISA resource name out=w538:refnum<visa-resource-name>, error out=w537:errorcluster)  [unwired: 1 out]
                }
                frame 2 {
                  # "Wavelength 2: 561 nm"
                  n89 = VISA Write(VISA resource name=w555, write buffer="7 1,3\r", error in (no error)=w554) -> (VISA resource name out=w551:refnum<visa-resource-name>, error out=w552:errorcluster)  [unwired: 1 out]
                  n90 = call-poly <vilib>:"DAQmx Write.vi"("task/channels in"=w548, "data"=bool[] [FALSE, FALSE, TRUE], "error in"=w547) -> ("task out"=w550:refnum<k21>, "error out"=w549:errorcluster)  [unwired: 10 in, 1 out]
                }
              }
              n91 = Divide(x=w492, y=2.0) -> (x/y=w489:dbl)
              n92 = Select(t=w489, s="Manual LCVR?", f=w490) -> (s? t:f=w488:dbl)
              "Output V" <- w488
              n93 = call-poly <vilib>:"DAQmx Write.vi"("task/channels in"=w514, "data"=w488, "error in"=w513) -> ("task out"=w512:refnum<k21>, "error out"=w511:errorcluster)  [unwired: 10 in, 1 out]
            }
            frame #2 {
              # "if it's the first frame in the sequence of SIM frames, does the stage need to move?"
              n94 = local read "Channels"() -> (w576:i16)
              n95 = local read "Positions"() -> (w565:i32)
              n96 = Greater?(x=w576, y=i16 1) -> (0:w575:bool)
              n97 = Greater?(x=w565, y=1) -> (0:w567:bool)
              n98 = And(x=w575, y=w568) -> (x .and. y?=w574:bool)
              n99 = And(x=w567, y=w568) -> (x .and. y?=w562:bool)
              n100 = case shown="True" w562 {
                tunnel: w564 -> [w594 w605]
                tunnel: w563 -> [w593 w604]
                tunnel: [w594 w602] -> w561
                tunnel: [w593 w601] -> w560
                tunnel: w559 -> [w592 w598]
                tunnel: w558 -> [w591 w597]
                tunnel: [w592 w596] -> w557
                tunnel: [w591 w595] -> w556
                frame False {
                }
                frame True {
                  n101 = local read "Pos N"() -> (w603:i32)
                  n102 = local read "First pos"() -> (w600:bool)
                  n103 = Not(x=w600) -> (.not. x?=w599:bool)
                  n104 = case shown="True" w599 {
                    tunnel: w605 -> [w610 w629]
                    tunnel: w604 -> [w609 w628]
                    tunnel: w603 -> [w612 w627]
                    tunnel: [w610 w626] -> w602
                    tunnel: [w609 w625] -> w601
                    tunnel: w598 -> [w607 w622]
                    tunnel: w597 -> [w606 w621]
                    tunnel: [w607 w618] -> w596
                    tunnel: [w606 w617] -> w595
                    frame False {
                      # "if we have just started the acquisition then don't move the stage, this will happen on the next SIM sequence for the next position"
                      n105 = Increment(x=w612) -> (x+1=w611:i32)
                      n106 = local write "First pos"(FALSE ("First pos")) -> ()
                      n107 = local write "Pos N"(w611) -> ()
                    }
                    frame True {
                      # "send TTL output to ASI control"
                      n108 = flat-sequence {
                        tunnel: w629 -> [w645]
                        tunnel: w628 -> [w644]
                        tunnel: w627 -> [w632]
                        tunnel: [w639] -> w624
                        tunnel: [w638] -> w623
                        tunnel: w622 -> [w637]
                        tunnel: w621 -> [w636]
                        tunnel: [w637] -> w620
                        tunnel: [w636] -> w619
                        tunnel: w624 -> [w651]
                        tunnel: w623 -> [w650]
                        tunnel: w620 -> [w649]
                        tunnel: w619 -> [w648]
                        tunnel: [w651] -> w616
                        tunnel: [w650] -> w615
                        tunnel: [w647] -> w614
                        tunnel: [w646] -> w613
                        tunnel: [w658] -> w617
                        tunnel: [w659] -> w618
                        tunnel: [w660] -> w625
                        tunnel: [w661] -> w626
                        tunnel: w616 -> [w661]
                        tunnel: w615 -> [w660]
                        tunnel: w614 -> [w659]
                        tunnel: w613 -> [w658]
                        frame #0 {
                          n109 = local read "Positions"() -> (w633:i32)
                          n110 = Increment(x=w632) -> (x+1=w631:i32)
                          n111 = call-poly <vilib>:"DAQmx Write.vi"("task/channels in"=w645, "data"=TRUE, "error in"=w644) -> ("task out"=w642:refnum<k21>, "error out"=w641:errorcluster)  [unwired: 10 in, 1 out]
                          n112 = Equal?(x=w633, y=w631) -> (x = y?=w630:bool)
                          n113 = local write "Last pos"(w630) -> ()
                          n114 = call-poly <vilib>:"DAQmx Write.vi"("task/channels in"=w642, "data"=FALSE, "error in"=w641) -> ("task out"=w639:refnum<k21>, "error out"=w638:errorcluster)  [unwired: 10 in, 1 out]
                          n115 = Select(t=0, s=w630, f=w631) -> (s? t:f=w635:i32)
                          n116 = local write "Pos N"(w635) -> ()
                        }
                        frame #1 {
                          # "wait until move complete"
                          n117 = while {
                            tunnel: w649 -> [w655]
                            tunnel: w648 -> [w654]
                            tunnel: [w653] -> w647
                            tunnel: [w652] -> w646
                            stop <- w656 stop-if-true
                            n118 = call-poly <vilib>:"DAQmx Read.vi"("task/channels in"=w655, "error in"=w654) -> ("task out"=w653:refnum<k21>, "data"=w656:bool, "error out"=w652:errorcluster)  [unwired: 11 in]
                          }
                        }
                        frame #2 {
                          # "let stage settle"
                          n119 = Wait (ms)(milliseconds to wait=u32 200) -> ()  [unwired: 1 out]
                        }
                      }
                    }
                  }
                }
              }
              n120 = case shown="True" w574 {
                tunnel: w572 -> [w663 w667]
                tunnel: w571 -> [w662 w666]
                tunnel: [w663 w665] -> w570
                tunnel: [w662 w664] -> w569
                frame False {
                }
                frame True {
                  n121 = local read "use z offset"() -> (w668:bool)
                  n122 = Wait (ms)(milliseconds to wait=u32 80) -> ()  [unwired: 1 out]
                  n123 = case shown="True" w668 {
                    tunnel: w667 -> [w671 w678]
                    tunnel: w666 -> [w670 w677]
                    tunnel: [w671 w676] -> w665
                    tunnel: [w670 w675] -> w664
                    frame False {
                    }
                    frame True {
                      n124 = local read "z offset (um)"() -> (w673:dbl)
                      n125 = call "Zpos to V.vi"(1:TRUE ("Z step?"), "Z (um)"=w673) -> ("V"=w674:dbl)  [unwired: 1 in]
                      n126 = call-poly <vilib>:"DAQmx Write.vi"("task/channels in"=w678, "data"=w674, "error in"=w677) -> ("task out"=w676:refnum<k21>, "error out"=w675:errorcluster)  [unwired: 10 in, 1 out]
                    }
                  }
                }
              }
            }
            frame #3 {
              n127 = call-poly <vilib>:"DAQmx Write.vi"("task/channels in"=w700, "data"=TRUE, "error in"=w699) -> ("task out"=w698:refnum<k21>, "error out"=w697:errorcluster)  [unwired: 10 in, 1 out]
            }
            frame #4 {
              n128 = local read "Exposure (ms)"() -> (w706:u32)
              n129 = Wait (ms)(milliseconds to wait=w706) -> ()  [unwired: 1 out]
            }
            frame #5 {
              n130 = call-poly <vilib>:"DAQmx Write.vi"("task/channels in"=w739, "data"=FALSE) -> ("task out"=w740:refnum<k21>)  [unwired: 11 in, 2 out]
            }
            frame #6 {
              n131 = while {
                tunnel: [w775] -> w768
                tunnel: w767 -> [w775]
                tunnel: [w774] -> w766
                tunnel: w765 -> [w774]
                tunnel: w764 -> [w773]
                tunnel: w763 -> [w772]
                tunnel: [w771] -> w762
                tunnel: [w770] -> w761
                stop <- w769 stop-if-true
                # "Wait until Trigger Ready received"
                n132 = call-poly <vilib>:"DAQmx Read.vi"("task/channels in"=w773, "error in"=w772) -> ("task out"=w770:refnum<k21>, "data"=w769:bool, "error out"=w771:errorcluster)  [unwired: 11 in]
              }
            }
            frame #7 {
              # "Switch off the laser"
              # "Post exposure tasks"
              n133 = local read "SIM \nFrames"() -> (w791:i16)
              n134 = local read "Channels"() -> (w790:i16)
              n135 = local read "# z steps"() -> (w788:i16)
              n136 = local read "Current Frame"() -> (w787:i32)
              n137 = Multiply(x=w791, y=w790) -> (x*y=w789:i16)
              n138 = Multiply(x=w788, y=w789) -> (x*y=w786:i16)
              n139 = Quotient & Remainder(x=w787, y=w786) -> (x-y*floor(x/y)=w785:i32)  [unwired: 1 out]
              n140 = Equal To 0?(x=w785) -> (x = 0?=w784:bool)
              n141 = call-poly <vilib>:"DAQmx Write.vi"("task/channels in"=w798, "data"=bool[] [FALSE, FALSE, FALSE], "error in"=w797) -> ()  [unwired: 10 in, 3 out]
              n142 = case shown="True" w794 {
                frame False {
                }
                frame True {
                  # "if it's the final frame, on the next frame move the z position"
                  n143 = local read "z #"() -> (w812:i16)
                  n144 = Increment(x=w812) -> (x+1=w811:i16)
                  n145 = local write "z #"(w811) -> ()
                  n146 = local write "Z move"(TRUE) -> ()
                }
              }
              n147 = local read "Interval"() -> (w800:u32)
              n148 = local read "Last pos"() -> (w778:bool)
              n149 = Not Equal To 0?(x=w800) -> (x != 0?=w799:bool)
              n150 = And(x=w794, y=w799) -> (x .and. y?=w783:bool)
              n151 = And(x=w783, y=w784) -> (x .and. y?=w777:bool)
              n152 = And(x=w777, y=w778) -> (x .and. y?=w776:bool)
              n153 = case shown="True" w776 {
                tunnel: w800 -> [_ w817]
                frame False {
                }
                frame True {
                  # "Wait for requested duration"
                  n154 = local read "Int unit"() -> (w818:enum16{"ms", "s", "min"})
                  n155 = call "Wait Interval.vi"("Interval unit"=w818, "Interval"=w817) -> ("Wait"=w815:u32)  [unwired: 9 in]
                  n156 = local write "Last pos"(FALSE ("Last pos")) -> ()
                  n157 = local write "Waiting"(TRUE ("Waiting")) -> ()
                  n158 = for {
                    N: w815 -> [w821]
                    i -> [w822]
                    n159 = Subtract(x=w821, y=w822) -> (x-y=w820:i32)
                    n160 = Divide(x=w820, y=1000) -> (x/y=w819:dbl)
                    n161 = local write "Time to next"(w819) -> ()
                    n162 = Wait (ms)(milliseconds to wait=u32 1) -> ()  [unwired: 1 out]
                  }
                }
              }
            }
          }
          n163 = Equal?(x=w248, y=w245) -> (x = y?=w247:bool)
          n164 = case shown="True" w247 {
            frame False {
            }
            frame True {
              n165 = local write "Auto Z"(FALSE ("Auto Z")) -> ()
            }
          }
        }
        n166 = local read "Piezo (um)"() -> (w184:dbl)
        n167 = control-ref of="Acquire"() -> (w237:refnum<vi>)
        n168 = control-ref of="Stop acq"() -> (w214:refnum<vi>)
        n169 = call-poly <vilib>:"DAQmx Write.vi"("task/channels in"=w207, "data"=FALSE, "error in"=w205) -> ("task out"=w206:refnum<k21>, "error out"=w204:errorcluster)  [unwired: 10 in, 1 out]
        n170 = local write "Waiting"(FALSE ("Waiting")) -> ()
        n171 = local write "Z move"(FALSE ("Z move")) -> ()
        n172 = VISA Close(VISA resource name=w209) -> ()  [unwired: 1 in, 1 out]
        n173 = call-poly <vilib>:"DAQmx Write.vi"("task/channels in"=w224, "data"=0.555, "error in"=w223) -> ("task out"=w222:refnum<k21>, "error out"=w221:errorcluster)  [unwired: 10 in, 1 out]
        n174 = property class="Bool (strict)"(reference=w237, "Value"=FALSE ("data")) -> ()  [unwired: 1 in, 2 out]
        n175 = property class="Bool (strict)"(reference=w214, "Value"=FALSE ("Visible")) -> ()  [unwired: 1 in, 2 out]
        n176 = call "Zpos to V.vi"(1:FALSE ("Z step?"), "Z (um)"=w184) -> ("V"=w182:dbl)  [unwired: 1 in]
        n177 = call-poly <vilib>:"DAQmx Write.vi"("task/channels in"=w190, "data"=w182, "error in"=w189) -> ("task out"=w188:refnum<k21>, "error out"=w187:errorcluster)  [unwired: 10 in, 1 out]
        n178 = Merge Errors(w232, w231, w221, w210) -> (w233:errorcluster)
        n179 = Unbundle By Name(w233) -> ("status"=w241:bool)
      }
      event "Live mode": Value Change {
        n180 = event-data() -> ("NewVal"=w828:bool)  [unwired: 1 in, 2 out]
        n181 = case shown="True" w828 {
          tunnel: w827 -> [_ w832]
          tunnel: [w829 w831] -> w826
          tunnel: w825 -> [w829 w830]
          frame False {
          }
          frame True {
            n182 = Enqueue Element(queue=w832, element=enum16{"Live", "Stop", "Acquire"}."Live", error in (no error)=w830) -> (error out=w831:errorcluster)  [unwired: 1 in, 2 out]
          }
        }
      }
      event "Manual DIO": Value Change {
        n183 = event-data() -> ()  [unwired: 1 in, 5 out]
        n184 = local read "Ch N"() -> (w834:T1)
        n185 = call "Channel ID to Wave ID.vi"("Ch N"=w834, "Channel ID"=i16 0) -> ("Wave ID"=w836:i16)  [unwired: 9 in]
        n186 = case shown="0, Default" w836 {
          tunnel: w838 -> [w843 w847 w851]
          tunnel: w837 -> [w842 w846 w850]
          tunnel: [w840 w845 w853] -> _
          tunnel: [w839 w844 w852] -> _
          frame 0, Default {
            # "Wavelength 0: 488nm"
            n187 = call-poly <vilib>:"DAQmx Write.vi"("task/channels in"=w843, "data"=bool[] [TRUE, FALSE, FALSE], "error in"=w842) -> ("task out"=w840:refnum<k21>, "error out"=w839:errorcluster)  [unwired: 10 in, 1 out]
          }
          frame 1 {
            # "Wavelength 1: 640nm"
            n188 = call-poly <vilib>:"DAQmx Write.vi"("task/channels in"=w847, "data"=bool[] [FALSE, TRUE, FALSE], "error in"=w846) -> ("task out"=w845:refnum<k21>, "error out"=w844:errorcluster)  [unwired: 10 in, 1 out]
          }
          frame 2 {
            # "Wavelength 2: 561 nm"
            n189 = call-poly <vilib>:"DAQmx Write.vi"("task/channels in"=w851, "data"=bool[] [FALSE, FALSE, TRUE], "error in"=w850) -> ("task out"=w853:refnum<k21>, "error out"=w852:errorcluster)  [unwired: 10 in, 1 out]
          }
        }
      }
      event "LCVR V": Value Change {
        n190 = event-data() -> ()  [unwired: 1 in, 5 out]
        n191 = Divide(x="LCVR V", y=2.0) -> (x/y=w854:dbl)
        n192 = local write "Output V"(w854) -> ()
        n193 = call-poly <vilib>:"DAQmx Write.vi"("task/channels in"=w858, "data"=w854, "error in"=w857) -> ()  [unwired: 10 in, 3 out]
      }
      event "Ch 0", "Ch 1", "Ch 2": Value Change {
        n194 = event-data() -> ()  [unwired: 1 in, 2 out]
        n195 = local read "Ch 0"() -> (w862:T2)
        n196 = local read "Ch 1"() -> (w861:T2)
        n197 = local read "Ch 2"() -> (w860:T2)
        n198 = Bundle("Ch 0"=w862, "Ch 1"=w861, "Ch 2"=w860) -> (w859:T3)  [unwired: 1 in]
        n199 = local write "Ch N"(w859) -> ()
      }
      event "Frames", "SIM \nFrames", "Channels", "Interval", "Int unit", "Exposure (ms)", "# z steps": Value Change {
        n200 = event-data() -> ()  [unwired: 1 in, 5 out]
        n201 = local read "SIM \nFrames"() -> (w881:i16)
        n202 = local read "Frames"() -> (w882:i16)
        n203 = local read "Channels"() -> (w879:i16)
        n204 = local read "SIM \nFrames"() -> (w877:i16)
        n205 = local read "Exposure (ms)"() -> (w878:u32)
        n206 = local read "Channels"() -> (w875:i16)
        n207 = local read "# z steps"() -> (w869:i16)
        n208 = local read "Interval"() -> (w874:u32)
        n209 = Multiply(x=w882, y=w881) -> (x*y=w880:i16)
        n210 = Multiply(x=w877, y=w878) -> (x*y=w876:u32)
        n211 = Multiply(x=w880, y=w879) -> (x*y=w870:i16)
        n212 = Multiply(x=w876, y=w875) -> (x*y=w873:u32)
        n213 = Multiply(x=w870, y=w869) -> (x*y=w868:i16)
        n214 = local read "Frames"() -> (w871:i16)
        n215 = Add(x=w873, y=w874) -> (x+y=w872:u32)
        n216 = local read "# z steps"() -> (w866:i16)
        n217 = local write "Total Frames"(w868) -> ()
        n218 = Multiply(x=w872, y=w871) -> (x*y=w867:u32)
        n219 = Multiply(x=w867, y=w866) -> (x*y=w865:u32)
        n220 = Divide(x=w865, y=u32 1000) -> (x/y=w863:dbl)
        n221 = local write "Duration (s)"(w863) -> ()
      }
      event "Piezo V": Value Change {
        n222 = event-data() -> ()  [unwired: 1 in, 5 out]
        n223 = local read "Piezo V"() -> (w883:dbl)
        n224 = call-poly <vilib>:"DAQmx Write.vi"("task/channels in"=w885, "data"=w883, "error in"=w884) -> ()  [unwired: 10 in, 3 out]
      }
      event "Auto Z": Value Change {
        n225 = event-data() -> ()  [unwired: 1 in, 5 out]
        n226 = flat-sequence {
          tunnel: w893 -> [w896]
          tunnel: w892 -> [w897]
          tunnel: w891 -> [w895]
          tunnel: [w895] -> w889
          tunnel: w888 -> [w894]
          tunnel: [w894] -> w886
          tunnel: [w902] -> w890
          tunnel: w889 -> [w902]
          tunnel: [w901] -> w887
          tunnel: w886 -> [w901]
          tunnel: w890 -> [w907]
          tunnel: w887 -> [w906]
          frame #0 {
            n227 = call-poly <vilib>:"DAQmx Read.vi"("task/channels in"=w896, "error in"=w897) -> ("data"=w898:dbl)  [unwired: 11 in, 2 out]
            n228 = call "VtoZ.vi"("Voltage IN"=w898) -> ("Zpos OUT (um)"=w899:dbl)
            n229 = local write "Piezo (um)"(w899) -> ()
          }
          frame #1 {
            n230 = local read "Auto Z"() -> (w900:bool)
            n231 = call "ASI_z_control onoff.vi"("Z control"=w900) -> ()  [unwired: 1 in]
          }
          frame #2 {
            n232 = local read "Piezo (um)"() -> (w905:dbl)
            n233 = call "Zpos to V.vi"(1:FALSE ("Z step?"), "Z (um)"=w905) -> ("V"=w904:dbl)  [unwired: 1 in]
            n234 = call-poly <vilib>:"DAQmx Write.vi"("task/channels in"=w907, "data"=w904, "error in"=w906) -> ()  [unwired: 10 in, 3 out]
          }
        }
      }
      event "Next Pos": Value Change {
        n235 = event-data() -> ()  [unwired: 1 in, 5 out]
        n236 = call-poly <vilib>:"DAQmx Write.vi"("task/channels in"=w913, "data"=TRUE, "error in"=w912) -> ("task out"=w910:refnum<k21>, "error out"=w909:errorcluster)  [unwired: 10 in, 1 out]
        n237 = call-poly <vilib>:"DAQmx Write.vi"("task/channels in"=w910, "data"=FALSE, "error in"=w909) -> ()  [unwired: 10 in, 3 out]
      }
    }
  }
  n238 = while "UI event Loop" {
    tunnel: w25 -> [w923]
    tunnel: w23 -> [w920]
    tunnel: w22 -> [w919]
    tunnel: w21 -> [w918]
    tunnel: w20 -> [w917]
    tunnel: w19 -> [w916]
    tunnel: w18 -> [w915]
    tunnel: [w914] -> _
    stop <- w921 stop-if-true
    n239 = Dequeue Element(queue=w923, error in (no error)=w920) -> (element=w922:enum16{"Live", "Stop", "Acquire"}, error out=w914:errorcluster)  [unwired: 1 in, 2 out]
    n240 = case shown="\"Live\", Default" w922 {
      tunnel: [w924 TRUE w933] -> w921
      tunnel: w919 -> [_ _ w932]
      tunnel: w918 -> [_ _ w931]
      tunnel: w917 -> [_ _ w930]
      tunnel: w916 -> [_ _ w929]
      tunnel: w915 -> [_ _ w928]
      frame "Acquire" {
        n241 = local read "Stop acq"() -> (w924:bool)
      }
      frame "Stop" {
      }
      frame "Live", Default {
        n242 = while {
          tunnel: w932 -> [w950]
          tunnel: w931 -> [w944]
          tunnel: w930 -> [w941]
          tunnel: w929 -> [w940]
          tunnel: w928 -> [w939]
          tunnel: [w938] -> w927
          stop <- w951 continue-if-true
          n243 = flat-sequence {
            tunnel: w944 -> [w960]
            tunnel: w950 -> [w961]
            tunnel: [w961] -> w943
            tunnel: [w960] -> w942
            tunnel: w941 -> [w958]
            tunnel: w940 -> [w957]
            tunnel: w939 -> [w955]
            tunnel: [w953] -> w934
            tunnel: [w982] -> w948
            tunnel: [w981] -> w945
            tunnel: w943 -> [w984]
            tunnel: w942 -> [w981]
            tunnel: [w980] -> w935
            tunnel: w934 -> [w980]
            tunnel: [w988] -> w949
            tunnel: w948 -> [w988]
            tunnel: [w987] -> w946
            tunnel: w945 -> [w987]
            tunnel: [w986] -> w936
            tunnel: w935 -> [w986]
            tunnel: w949 -> [w992]
            tunnel: [w990] -> w947
            tunnel: w946 -> [w990]
            tunnel: [w989] -> w937
            tunnel: w936 -> [w989]
            tunnel: w947 -> [w995]
            tunnel: [w994] -> w938
            tunnel: w937 -> [w994]
            frame #0 {
              n244 = local read "Ch N"() -> (w959:T1)
              n245 = call "Channel ID to Wave ID.vi"("Ch N"=w959, "Channel ID"=i16 0) -> ("Wave ID"=w956:i16)  [unwired: 9 in]
              n246 = case shown="2" w956 {
                tunnel: w958 -> [w967 w972 w975]
                tunnel: [w965 w971 w976] -> _
                tunnel: w957 -> [w964 w970 w979]
                tunnel: [w962 w969 w977] -> _
                frame 0, Default {
                  # "Wavelength 0: 488nm"
                  n247 = VISA Write(VISA resource name=w964, write buffer="7 1,4\r") -> (VISA resource name out=w962:refnum<visa-resource-name>)  [unwired: 1 in, 2 out]
                  n248 = call-poly <vilib>:"DAQmx Write.vi"("task/channels in"=w967, "data"=bool[] [TRUE, FALSE, FALSE]) -> ("task out"=w965:refnum<k21>)  [unwired: 11 in, 2 out]
                }
                frame 1 {
                  # "Wavelength 1: 640nm"
                  n249 = call-poly <vilib>:"DAQmx Write.vi"("task/channels in"=w972, "data"=bool[] [FALSE, TRUE, FALSE]) -> ("task out"=w971:refnum<k21>)  [unwired: 11 in, 2 out]
                  n250 = VISA Write(VISA resource name=w970, write buffer="7 1,2\r") -> (VISA resource name out=w969:refnum<visa-resource-name>)  [unwired: 1 in, 2 out]
                }
                frame 2 {
                  # "Wavelength 2: 561 nm"
                  n251 = VISA Write(VISA resource name=w979, write buffer="7 1,3\r") -> (VISA resource name out=w977:refnum<visa-resource-name>)  [unwired: 1 in, 2 out]
                  n252 = call-poly <vilib>:"DAQmx Write.vi"("task/channels in"=w975, "data"=bool[] [FALSE, FALSE, TRUE]) -> ("task out"=w976:refnum<k21>)  [unwired: 11 in, 2 out]
                }
              }
              n253 = local write "Ch"(w956) -> ()
              n254 = call-poly <vilib>:"DAQmx Write.vi"("task/channels in"=w955, "data"=TRUE) -> ("task out"=w953:refnum<k21>)  [unwired: 11 in, 2 out]
            }
            frame #1 {
              n255 = call-poly <vilib>:"DAQmx Write.vi"("task/channels in"=w984, "data"=TRUE) -> ("task out"=w982:refnum<k21>)  [unwired: 11 in, 2 out]
            }
            frame #2 {
              n256 = local read "Exposure (ms)"() -> (w985:u32)
              n257 = Wait (ms)(milliseconds to wait=w985) -> ()  [unwired: 1 out]
            }
            frame #3 {
              n258 = call-poly <vilib>:"DAQmx Write.vi"("task/channels in"=w992, "data"=FALSE) -> ()  [unwired: 11 in, 3 out]
            }
            frame #4 {
              n259 = Tick Count (ms)() -> (millisecond timer value=w993:u32)
              n260 = while {
                tunnel: [w1004] -> _
                tunnel: w995 -> [w1003]
                tunnel: w993 -> [w1002]
                stop <- w997 stop-if-true
                # "Wait until Trigger Ready received"
                n261 = Tick Count (ms)() -> (millisecond timer value=w1001:u32)
                n262 = call-poly <vilib>:"DAQmx Read.vi"("task/channels in"=w1003) -> ("task out"=w1004:refnum<k21>, "data"=w998:bool)  [unwired: 12 in, 1 out]
                n263 = Subtract(x=w1001, y=w1002) -> (x-y=w1000:u32)
                n264 = Greater?(x=w1000, y=u32 5000) -> (0:w999:bool)
                n265 = Or(x=w998, y=w999) -> (x .or. y?=w997:bool)
              }
            }
          }
          n266 = local read "Live mode"() -> (w951:bool)
        }
        n267 = call-poly <vilib>:"DAQmx Write.vi"("task/channels in"=w927, "data"=TRUE) -> ()  [unwired: 11 in, 3 out]
        n268 = local read "Stop acq"() -> (w933:bool)
      }
    }
  }
  n269 = call <vilib>:"DAQmx Clear Task.vi"("task in"=w2, "error in"=w1) -> ("error out"=w3:errorcluster)  [unwired: 13 in]
  n270 = call <vilib>:"DAQmx Clear Task.vi"("task in"=w13, "error in"=w12) -> ("error out"=w11:errorcluster)  [unwired: 13 in]
  n271 = call <vilib>:"DAQmx Clear Task.vi"("task in"=w7, "error in"=w6) -> ("error out"=w8:errorcluster)  [unwired: 13 in]
  n272 = Release Queue(queue=w25, error in (no error)=w24) -> ()  [unwired: 1 in, 3 out]
  n273 = call <vilib>:"DAQmx Clear Task.vi"("task in"=w46, "error in"=w44) -> ("error out"=w38:errorcluster)  [unwired: 13 in]
  n274 = call <vilib>:"DAQmx Clear Task.vi"("task in"=w41, "error in"=w42) -> ("error out"=w37:errorcluster)  [unwired: 13 in]
  n275 = call <vilib>:"DAQmx Clear Task.vi"("task in"=w31, "error in"=w29) -> ("error out"=w30:errorcluster)  [unwired: 13 in]
  n276 = call <vilib>:"DAQmx Clear Task.vi"("task in"=w35, "error in"=w34) -> ("error out"=w32:errorcluster)  [unwired: 13 in]
  n277 = Merge Errors(w38, w37, w30, w32, w11, w8, w3) -> (w36:errorcluster)
  n278 = call <vilib>:"Simple Error Handler.vi"("error in (no error)"=w36) -> ()  [unwired: 4 in, 5 out]
